vi "sub_Chop_Packet.vi"(6 "bin_size":i32=16, 9 "Energy Threshold":dbl=1e-05, 11 "Input Complex Samples":cdb[](array[numeric])) -> (2 "Packet Detection Error?":bool, 3 "packet_arr":cdb[][](array[numeric]))   [LabVIEW 2015]
panel:
  in  "Use stored data?":bool
  out "Thresholded Signal":bool[](array[boolean])
  out "Averaged Power Signal":dbl[](array[numeric])
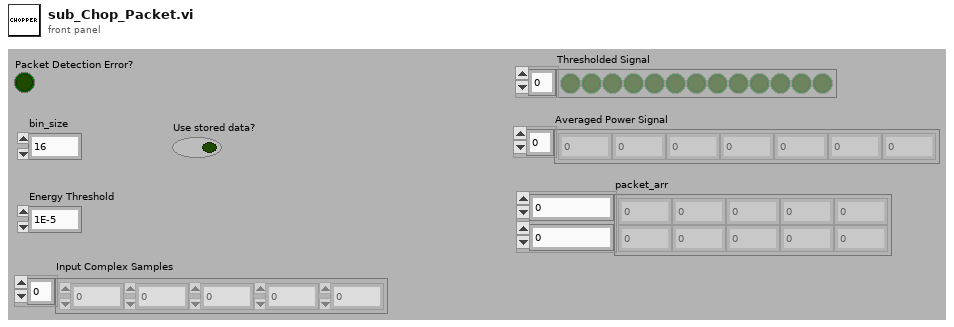
[diagram p1: front panel]
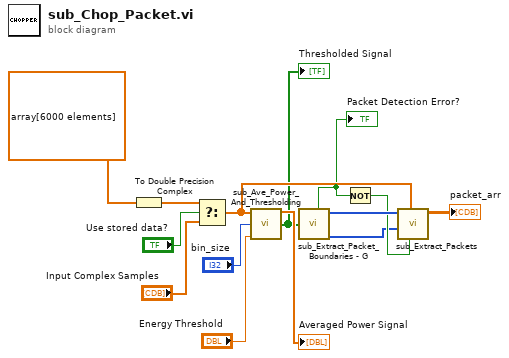
[diagram p0: block diagram]
diagram:
  n1 = To Double Precision Complex(1:dbl[] array[6000 elements] ("Received Signal")) -> (0:w14:cdb[])
  n2 = Select(t=w14, s="Use stored data?", f="Input Complex Samples") -> (s? t:f=w8:cdb[])
  n3 = call "sub_Ave_Power_And_Thresholding.vi"("Input Complex Samples"=w8, "bin_size"="bin_size", "threshold"="Energy Threshold") -> ("Averaged Power Signal"=→"Averaged Power Signal":dbl[], "Thresholded Signal"=w2:bool[])  [unwired: 11 in]
  "Thresholded Signal" <- w2
  n4 = call "sub_Extract_Packet_Boundaries - G.vi"("Thresholded Signal"=w2) -> ("packet_start_loc"=w9:i32[], "packet_end_loc"=w1:i32[], "Packet Detection Error?"=w5:bool)  [unwired: 2 in]
  "Packet Detection Error?" <- w5
  n5 = Not(x=w5) -> (.not. x?=w4:bool)
  n6 = call "sub_Extract_Packets.vi"("Enable?"=w4, "Input Complex Samples"=w8, "packet_end_loc"=w1, "packet_start_loc"=w9) -> ("packet_arr"=→"packet_arr":cdb[][])  [unwired: 7 in]
